vi "daqCtrl.vi"(9 "rate":dbl=1000.0 format="%0.2f", 10 "data":dbl[][](array[numeric]) format="%0.2f", 11 "Channels":string[](array[string])) -> (0 "error out":errorcluster)   [LabVIEW 2017]
uses:
  <vilib>/DAQmx/write.llb/DAQmx Write (Analog 2D DBL NChan NSamp).vi
  <vilib>/DAQmx/create/channels.llb/DAQmx Create Channel (AO-Voltage-Basic).vi
  <vilib>/DAQmx/configure/timing.llb/DAQmx Timing (Sample Clock).vi
  <vilib>/DAQmx/miscellaneous.llb/DAQmx Fill In Error Info.vi
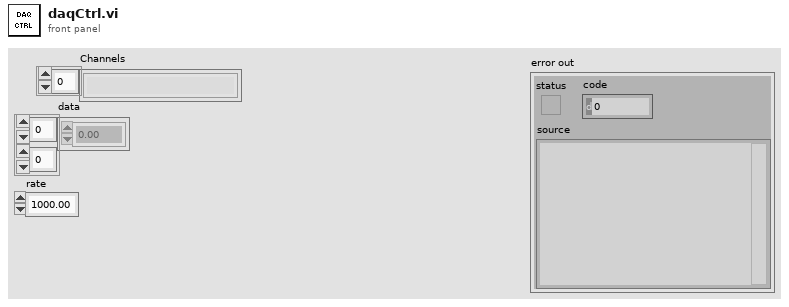
[diagram p1: front panel]
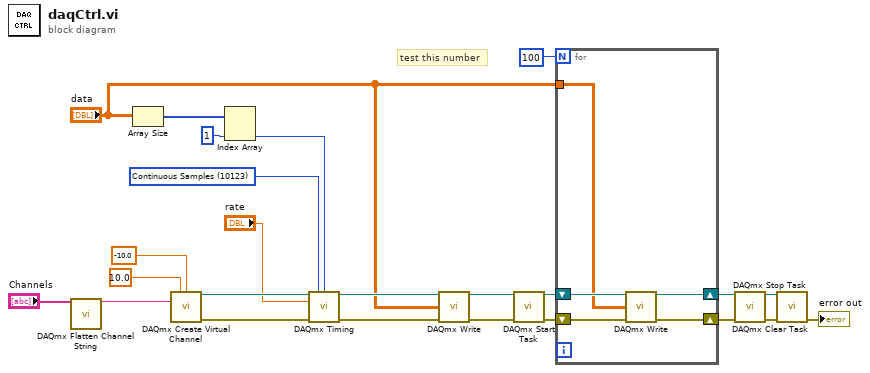
[diagram p0: block diagram]
diagram:
  w3 = 10123 items=["Finite Samples"=10178, "Continuous Samples"=10123, "Hardware Timed Single Point"=12522] ("sample mode")
  # "test this number"
  n1 = call <vilib>:"DAQmx Flatten Channel String.vi"("names in"="Channels") -> ("names out"=w20:string)  [unwired: 13 in, 1 out]
  n2 = Array Size(array="data") -> (size(s)=w6:i32[])
  n3 = call-poly <vilib>:"DAQmx Create Virtual Channel.vi"("maximum value"=10.0, "minimum value"=-10.0, "physical channels"=w20) -> ("task out"=w11:refnum<k21>, "error out"=w12:errorcluster)  [unwired: 11 in]
  n4 = Index Array(array=w6, index #2=1 ("index")) -> (element #2=w4:i32)  [unwired: 1 in, 1 out]
  n5 = call-poly <vilib>:"DAQmx Timing.vi"("task/channels in"=w11, "sample mode"=w3, "samples per channel"=w4, "rate"="rate", "error in"=w12) -> ("task out"=w14:refnum<k21>, "error out"=w13:errorcluster)  [unwired: 9 in]
  n6 = call-poly <vilib>:"DAQmx Write.vi"("task/channels in"=w14, "data"="data", "error in"=w13) -> ("task out"=w9:refnum<k21>, "error out"=w8:errorcluster)  [unwired: 10 in, 1 out]
  n7 = call <vilib>:"DAQmx Start Task.vi"("task/channels in"=w9, "error in"=w8) -> ("task out"=w16:refnum<k21>, "error out"=w15:errorcluster)  [unwired: 12 in]
  n8 = for {
    N: 100 -> [_]
    shift-right: [w29] -> w2
    shift-left: w16 -> [w27]
    shift-right: [w28] -> w1
    shift-left: w15 -> [w26]
    tunnel: "data" -> [w25]
    n9 = call-poly <vilib>:"DAQmx Write.vi"("task/channels in"=w27, "data"=w25, "error in"=w26) -> ("task out"=w29:refnum<k21>, "error out"=w28:errorcluster)  [unwired: 10 in, 1 out]
  }
  n10 = call <vilib>:"DAQmx Stop Task.vi"("task/channels in"=w2, "error in"=w1) -> ("task out"=w18:refnum<k21>, "error out"=w17:errorcluster)  [unwired: 12 in]
  n11 = call <vilib>:"DAQmx Clear Task.vi"("task in"=w18, "error in"=w17) -> ("error out"=→"error out":errorcluster)  [unwired: 13 in]
